vi "generate_error.vi"(6 "show call chain? (T)":bool=TRUE, 8 "error in (no error)":errorcluster, 10 "Data":variant, 11 "error":T1) -> (0 "error out":errorcluster)   [LabVIEW 2015, in "lv-bin-wget.lvlib"]
uses:
  lv-bin-wget.lvlib
  _controls/error.ctl
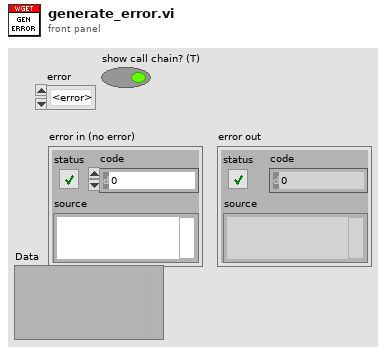
[diagram p1: front panel]
types:
  T1 = typedef "lv-bin-wget.lvlib/error.ctl" = enum16{"<error>", "wget_x86_missing", "wget_x64_missing"}
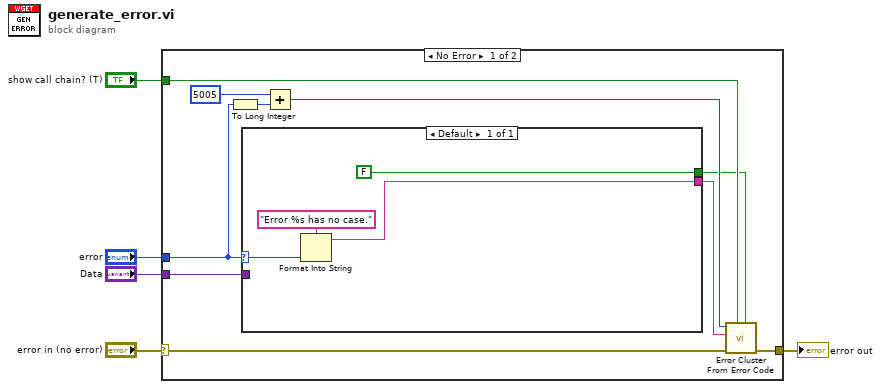
[diagram p0: block diagram]
diagram:
  n1 = case shown="No Error" "error in (no error)" {
    selector: "error in (no error)" -> [w6 w20]
    tunnel: "Data" -> [w15 _]
    tunnel: [w14 w20] -> w3
    tunnel: "error" -> [w12 _]
    tunnel: "show call chain? (T)" -> [w8 _]
    frame No Error {
      n2 = To Long Integer(number=w12) -> (32bit integer=w11:i32)
      n3 = case shown="Default" w12 {
        selector: w12 -> [w18]
        tunnel: w15 -> [_]
        tunnel: [w17] -> w9
        tunnel: [FALSE] -> w7
        frame Default {
          n4 = Format Into String(format string="Error %s has no case.", w18) -> (resulting string=w17:string)  [unwired: 2 in, 1 out]
        }
      }
      n5 = Add(x=5005, y=w11) -> (x+y=w10:i32)
      n6 = call <vilib>:"Error Cluster From Error Code.vi"("is warning? (False)"=w7, "show call chain? (False)"=w8, "error in (no error)"=w6, "error message (\"\")"=w9, "error code (0)"=w10) -> ("error out"=w14:errorcluster)  [unwired: 4 in]
    }
    frame Error {
    }
  }
  "error out" <- w3
